vi "case structure.vi"() -> ()   [LabVIEW 2020]
panel:
  out "result":bool
  in  "b":bool
  in  "a":bool
  in  "Boolean":bool
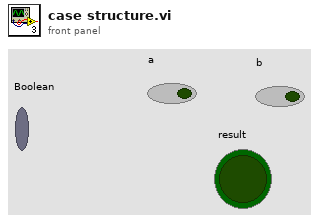
[diagram p1: front panel]
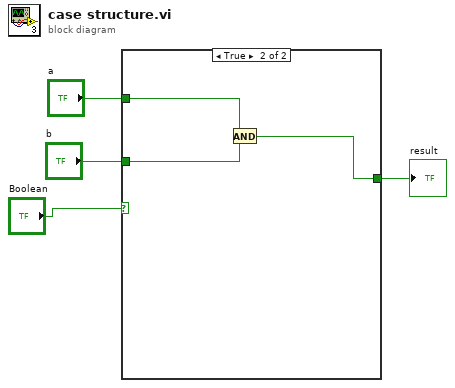
[diagram p0: block diagram]
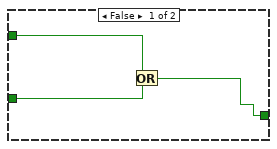
[diagram p2: hidden frame]
diagram:
  n1 = case shown="True" "Boolean" {
    tunnel: "a" -> [w7 w10]
    tunnel: "b" -> [w6 w9]
    tunnel: [w5 w8] -> w1
    frame False {
      n2 = Or(x=w7, y=w6) -> (x .or. y?=w5:bool)
    }
    frame True {
      n3 = And(x=w10, y=w9) -> (x .and. y?=w8:bool)
    }
  }
  "result" <- w1
